vi "Read All Card and Chnl Names.vi"(8 "error in (no error)":errorcluster, 11 "BME_DG_System in":refnum<class "BME_DG_System.lvclass">) -> (0 "error out":errorcluster, 1 "ChnlNames":string[](array[string]), 2 "CardNames":string[](array[string]), 3 "BME_DG_System out":refnum<class "BME_DG_System.lvclass">)   [LabVIEW 2009, in "POLARIS BME DG.lvlib" / "BME_DG_System.lvclass"]
uses:
  BME_DG_System.lvclass
  BME_DG_System.lvclass/BME_DG_System.ctl
  BME_DG_Base/BME_DG_Base.lvclass
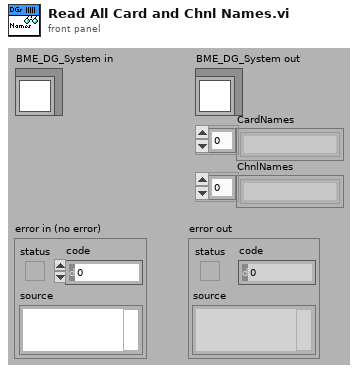
[diagram p1: front panel]
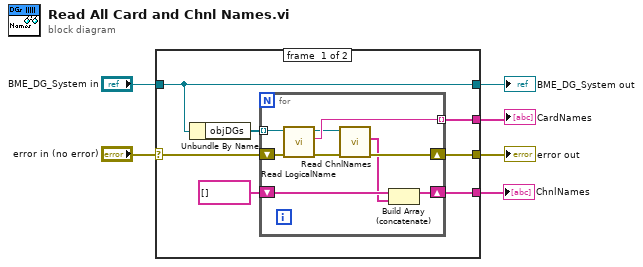
[diagram p0: block diagram]
diagram:
  n1 = case shown="No Error" "error in (no error)" {
    selector: "error in (no error)" -> [w10 w24]
    tunnel: [w9 w24] -> w5
    tunnel: [w13 w23] -> w3
    tunnel: "BME_DG_System in" -> [w13 w23]
    tunnel: [w11 _] -> w2
    tunnel: [w8 _] -> w1
    frame #0 {
      n2 = Unbundle By Name(w13) -> ("objDGs"=w12:refnum<class "BME_DG_Base.lvclass">[])
      n3 = for {
        tunnel: w12 -> [w22] mode=indexing
        tunnel: [w21] -> w11 mode=indexing
        shift-right: [w17] -> w9
        shift-left: w10 -> [w20]
        shift-right: [w14] -> w8
        shift-left: string[] [] -> [w16]
        n4 = call "Read LogicalName.vi"("error in (no error)"=w20, "BME_DG_Base in"=w22) -> ("error out"=w18:errorcluster, "LogicalName"=w21:string, "BME_DG_Base out"=w19:refnum<class "BME_DG_Base.lvclass">)  [unwired: 7 in]
        n5 = call-dynamic "Read ChnlNames.vi"("error in (no error)"=w18, "BME_DG_Base in"=w19) -> ("error out"=w17:errorcluster, "ChnlNames"=w15:string[])  [unwired: 7 in, 1 out]
        n6 = Build Array (concatenate)(w16, w15) -> (w14:string[])
      }
    }
    frame #1 {
    }
  }
  "error out" <- w5
  "BME_DG_System out" <- w3
  "CardNames" <- w2
  "ChnlNames" <- w1
